vi "Pasco Turn Shoot.vi"(0 "time/distance":dbl, 1 "desired heading":dbl, 2 "array index":i32, 3 "Misc4 IN":dbl, 4 "Misc3 IN":dbl, 5 "Misc2 IN":dbl, 6 "primitive time":i32, 7 "Misc1 IN":dbl) -> (16 "array index":i32, 17 "Misc1  OUT":dbl, 18 "Misc2 OUT":dbl, 19 "Misc4 OUT":dbl)   [LabVIEW 2011]
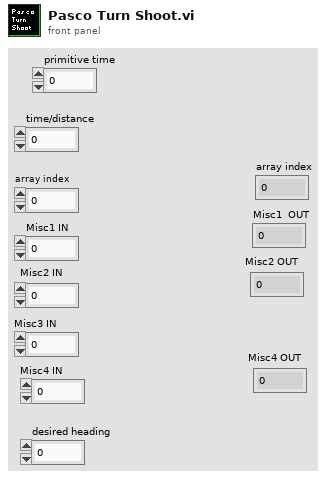
[diagram p1: front panel]
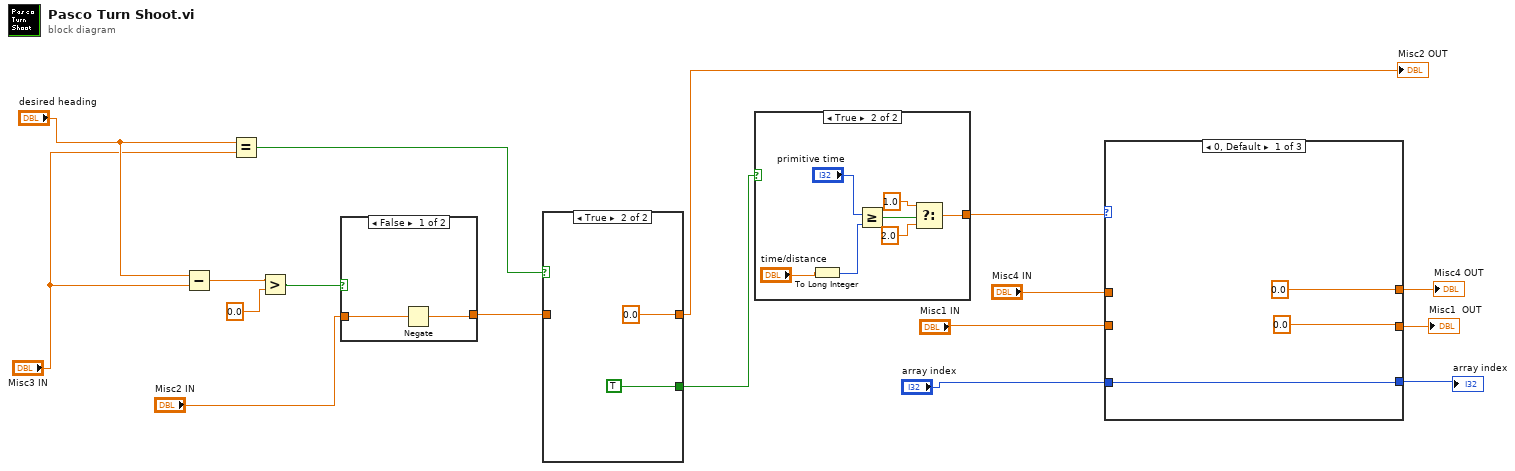
[diagram p0: block diagram]
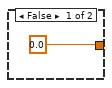
[diagram p2: hidden frame]
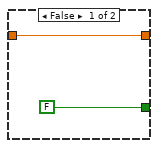
[diagram p3: hidden frame]
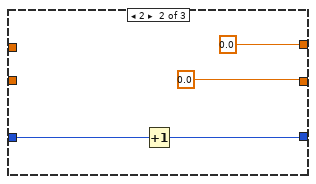
[diagram p5: hidden frame]
diagram:
  n1 = Subtract(x="desired heading", y="Misc3 IN") -> (x-y=w12:dbl)
  n2 = Equal?(x="desired heading", y="Misc3 IN") -> (x = y?=w16:bool)
  n3 = Greater?(x=w12, y=0.0) -> (0:w13:bool)
  n4 = case shown="False" w13 {
    tunnel: [w18 w20] -> w15
    tunnel: "Misc2 IN" -> [w19 w20]
    frame False {
      n5 = Negate(x=w19) -> (-x=w18:dbl)
    }
    frame True {
    }
  }
  n6 = case shown="True" w16 {
    tunnel: [w22 0.0] -> w3
    tunnel: w15 -> [w22 _]
    tunnel: [FALSE TRUE] -> w7
    frame False {
    }
    frame True {
    }
  }
  "Misc2 OUT" <- w3
  n7 = case shown="True" w7 {
    tunnel: [0.0 w30] -> w6
    frame False {
    }
    frame True {
      n8 = To Long Integer(number="time/distance") -> (32bit integer=w27:i32)
      n9 = Greater Or Equal?(x="primitive time", y=w27) -> (x >= y?=w31:bool)
      n10 = Select(t=1.0, s=w31, f=2.0) -> (s? t:f=w30:dbl)
    }
  }
  n11 = case shown="0, Default" w6 {
    tunnel: [0.0 0.0 w41] -> w4
    tunnel: "Misc1 IN" -> [_ _ w41]
    tunnel: "array index" -> [w34 w38 w42]
    tunnel: [w34 w37 w42] -> w5
    tunnel: [0.0 0.0 w40] -> w2
    tunnel: "Misc4 IN" -> [_ _ w40]
    frame 0, Default {
    }
    frame 2 {
      n12 = Increment(x=w38) -> (x+1=w37:i32)
    }
    frame 1 {
    }
  }
  "array index" <- w5
  "Misc1  OUT" <- w4
  "Misc4 OUT" <- w2
